vi "BLT Control Panel.vi"() -> ()   [LabVIEW 2018]
uses:
  Type Defs/Sensor Data.ctl
  Type Defs/Boxcar.ctl
panel:
  out "COPV PT":string="-123.37 lbf"
  in  "Data Log Button 2":bool
  out "LOX":dbl(slide) scale=0.0..90.0
  out "current time":timestamp=timestamp(3662240982.153583 s since 1904-01-01)
  out "loadcell 0":string="2.15 On/Off"
  out "loadcell 1":string="-119.97 On/Off"
  out "FUEL MV PT":string="-38.12 "
  out "LOX MV PT":string="-39.05 "
  out "loadcell 2":string="-359.34 On/Off"
  out "90%":string="15.79 °C"
  in  "Box cooler":bool
  out "NewVal":bool
  out "Ready To Fire Flag":bool
  out "Firing State":string[](array[string])=["System Is Not Armed", "  \n", " ", " ", " ", " ", " ", " "]
  in  "Arm Flag":bool
  in  "Sample Rate (secs)":u32=100
  out "Burn Time\nCountdown (secs)":string="0.00"
  out "Boxcar Data":T1={"AI Sensor Data"={"Sensor Array"=[{"Description"="P2 - LOX Tank Pressure", "Last Reading"="-124.93", "Coefs"=[-124.82, 244.17], "Eng Units"="psig"}, {"Description"="P3 - Fuel Tank Pressure", "Last Reading"="-124.93", "Coefs"=[-124.82, 244.17], "Eng Units"="psig"}, {"Description"="P1 - Chamber Pressure", "Last Reading"="-63.48", "Coefs"=[-63.442, 124.53], "Eng Units"="psig"}, {"Description"="Not Used", "Last Reading"="0.00", "Coefs"=[0.0, 0.0], "Eng Units"="psig"}, {"Description"="P5- DOME Reg.", "Last Reading"="-65.08", "Coefs"=[-65.132, -121.72], "Eng Units"="psig"}, {"Description"="Not Use", "Last Reading"="0.00", "Coefs"=[0.0, 0.0], "Eng Units"="psig"}, {"Description"="Load Cell", "Last Reading"="-5.17", "Coefs"=[-8.51, -8297.0], "Eng Units"="lb"}, {"Description"="P7 - Gnd High Pressure", "Last Reading"="-4.44", "Coefs"=[0.0, 10000.0], "Eng Units"="psig"}, {"Description"="High Press PT", "Last Reading"="20.64", "Coefs"=[-546.67, 1244.7], "Eng Units"="psig"}, {"Description"="Dome Reg PT", "Last Reading"="1.90", "Coefs"=[-126.3, 250.5], "Eng Units"="psig"}, {"Description"="FUEL PT", "Last Reading"="1.22", "Coefs"=[-134.15, 250.329], "Eng Units"=""}, {"Description"="LOX PT", "Last Reading"="1.10", "Coefs"=[-129.5, 251.22], "Eng Units"=""}, {"Description"="Chamber PT", "Last Reading"="1.05", "Coefs"=[-63.442, 124.53], "Eng Units"=""}, {"Description"="LOX MV PT", "Last Reading"="-39.05", "Coefs"=[-63.711, 124.59], "Eng Units"=""}, {"Description"="FUEL MV PT", "Last Reading"="-38.12", "Coefs"=[-62.615, 123.79], "Eng Units"=""}, {"Description"="", "Last Reading"="0.00", "Coefs"=[0.0, 0.0], "Eng Units"=""}, {"Description"="", "Last Reading"="2.15", "Coefs"=[1.9166, -16831.0], "Eng Units"="On/Off"}, {"Description"="Load Cell 0", "Last Reading"="-115.96", "Coefs"=[1.9166, -16831.0], "Eng Units"="On/Off"}, {"Description"="Load Cell 1", "Last Reading"="-318.18", "Coefs"=[-0.842, -16966.0], "Eng Units"="On/Off"}, {"Description"="Load Cell 2", "Last Reading"="3.51", "Coefs"=[-0.842, -16966.0], "Eng Units"="On/Off"}, {"Description"="Load Cell 1 - Veh Gross Weight", "Last Reading"="-123.37", "Coefs"=[-122.0, 8333.3], "Eng Units"="lbf"}, {"Description"="Load Cell 2 - - Veh Gross Weight", "Last Reading"="-1.64", "Coefs"=[0.0, 8333.33], "Eng Units"="lbf"}, {"Description"="Extra PT", "Last Reading"="-72.27", "Coefs"=[-72.241, 126.92], "Eng Units"=""}, {"Description"="Not Used", "Last Reading"="0.00", "Coefs"=[0.0, 0.0], "Eng Units"=""}, {"Description"="P6 - GHE Fill Pressure", "Last Reading"="-13651.00", "Coefs"=[-1035.0, 1261.6], "Eng Units"="psi"}, {"Description"="", "Last Reading"="0.00", "Coefs"=[], "Eng Units"=""}, {"Description"="", "Last Reading"="0.00", "Coefs"=[], "Eng Units"=""}, {"Description"="", "Last Reading"="0.00", "Coefs"=[], "Eng Units"=""}, {"Description"="", "Last Reading"="0.00", "Coefs"=[], "Eng Units"=""}, {"Description"="", "Last Reading"="0.00", "Coefs"=[], "Eng Units"=""}, {"Description"="", "Last Reading"="0.00", "Coefs"=[], "Eng Units"=""}, {"Description"="", "Last Reading"="0.00", "Coefs"=[], "Eng Units"=""}]}, "TC Array"=[15.7913203265, 15.7913203265, 15.7913203265, 15.7913203265, 15.7913203265, 15.7913203265, 15.7913203265, 1369.6815, 1369.6815, 1369.6815, 1369.6815, 1369.6815, 1369.6815, 1369.6815]}
  out "?":string="20.64 psig"
  out "Log Refnum":refnum<file>
  out "Log Epoch":u32=140317755
  out "Log Number":i32=426
  in  "Data Log Flag":bool
  out "File Path":path=path "C:/Users/Beach Launch Team/Desktop/EGSE/DATA LOGS/Default Log"
  out "Eng Data & Units":string[](array[string])=["-124.93 psig", "-124.94 psig", "-63.48 psig", "0.00 psig", "-65.08 psig", "0.00 psig", "-5.17 lb", "-4.44 psig", "20.64 psig", "1.90 psig", "1.22 ", "1.10 ", "1.05 ", "-39.05 ", "-38.12 ", "0.00 ", "2.15 On/Off", "-119.97 On/Off", "-359.34 On/Off", "3.51 On/Off", "-123.37 lbf", "-1.64 lbf", "-72.27 ", "0.00 ", "-13651.00 psi", "0.00 ", "0.00 ", "0.00 ", "0.00 ", "0.00 ", "0.00 ", "0.00 "]
  out "TC String Array":string[](array[string])=["15.79 °C", "15.79 °C", "15.79 °C", "15.79 °C", "15.79 °C", "15.79 °C", "15.79 °C", "1369.68 °C", "1369.68 °C", "1369.68 °C", "1369.68 °C", "1369.68 °C", "1369.68 °C", "1369.68 °C"]
  in  "Data Log Button":bool
  in  "Sequence Abort":bool
  out "Igniter Abort":bool
  out "Elapsed Time":u32=10552
  in  "Auto Sequence":bool
  in  "Auto Sequence Flag":bool
  out "Epoch":u32=136578
  out "Countdown (secs)":i32
  in  "MV Open Start":dbl
  in  "Burn Time":dbl=90.0
  in  "Igniter Start":dbl=-6.0
  in  "Countdown":dbl=-10.0
  in  "Igniter Minimum\nTemp (°C)":dbl=60.0
  in  "Auto Switch":bool=TRUE
  out "?":string="1369.68 °C"
  out "Thermometer 2":dbl(slide)=1369.6815 scale=0.0..1000.0
  out "Thermometer":dbl(slide)=1369.6815 scale=0.0..1000.0
  out "Igniter Temp (°C)":string="1369.68 °C"
  out "10%":string="15.79 °C"
  out "50%":string="15.79 °C"
  out "QD Sep Indicator":bool
  out "Liftoff Indicator":bool
  out "MV Closed Ind":bool
  out "MV Open Ind":bool
  out "?":string="1.90 psig"
  out "?":string="-4.44 psig"
  out "Dome Reg PT":string="1.90 psig"
  out "?":string="20.64 psig"
  out "Main Valve PT":string="1.05 "
  out "Fuel PT":string="1.22 "
  in  "High Press":bool
  in  "High Press Vent":bool
  in  "MV Open":bool
  in  "MV Closed":bool
  out "Lox PT":string="1.10 "
  in  "Remote QD Sep":bool
  in  "GHe Fill":bool
  in  "Igniter Pwr":bool
  in  "Dome Reg":bool
  in  "Dome Vent":bool
  in  "Fuel Vent":bool
  in  "LOX Vent":bool
  out "Relay States":bool[](array[boolean])
  in  "stop":bool
  in  "AI Sensor Data":T2={"Sensor Array"=[{"Description"="P2 - LOX Tank Pressure", "Last Reading"="-124.93", "Coefs"=[-124.82, 244.17], "Eng Units"="psig"}, {"Description"="P3 - Fuel Tank Pressure", "Last Reading"="-124.94", "Coefs"=[-124.82, 244.17], "Eng Units"="psig"}, {"Description"="P1 - Chamber Pressure", "Last Reading"="-63.48", "Coefs"=[-63.442, 124.53], "Eng Units"="psig"}, {"Description"="Not Used", "Last Reading"="0.00", "Coefs"=[0.0, 0.0], "Eng Units"="psig"}, {"Description"="P5- DOME Reg.", "Last Reading"="-65.08", "Coefs"=[-65.132, -121.72], "Eng Units"="psig"}, {"Description"="Not Use", "Last Reading"="0.00", "Coefs"=[0.0, 0.0], "Eng Units"="psig"}, {"Description"="Load Cell", "Last Reading"="-5.17", "Coefs"=[-8.51, -8297.0], "Eng Units"="lb"}, {"Description"="P7 - Gnd High Pressure", "Last Reading"="-4.44", "Coefs"=[0.0, 10000.0], "Eng Units"="psig"}, {"Description"="High Press PT", "Last Reading"="20.64", "Coefs"=[-546.67, 1244.7], "Eng Units"="psig"}, {"Description"="Dome Reg PT", "Last Reading"="1.90", "Coefs"=[-126.3, 250.5], "Eng Units"="psig"}, {"Description"="FUEL PT", "Last Reading"="1.22", "Coefs"=[-134.15, 250.329], "Eng Units"=""}, {"Description"="LOX PT", "Last Reading"="1.10", "Coefs"=[-129.5, 251.22], "Eng Units"=""}, {"Description"="Chamber PT", "Last Reading"="1.05", "Coefs"=[-63.442, 124.53], "Eng Units"=""}, {"Description"="LOX MV PT", "Last Reading"="-39.05", "Coefs"=[-63.711, 124.59], "Eng Units"=""}, {"Description"="FUEL MV PT", "Last Reading"="-38.12", "Coefs"=[-62.615, 123.79], "Eng Units"=""}, {"Description"="", "Last Reading"="0.00", "Coefs"=[0.0, 0.0], "Eng Units"=""}, {"Description"="", "Last Reading"="2.15", "Coefs"=[1.9166, -16831.0], "Eng Units"="On/Off"}, {"Description"="Load Cell 0", "Last Reading"="-119.97", "Coefs"=[1.9166, -16831.0], "Eng Units"="On/Off"}, {"Description"="Load Cell 1", "Last Reading"="-359.34", "Coefs"=[-0.842, -16966.0], "Eng Units"="On/Off"}, {"Description"="Load Cell 2", "Last Reading"="3.51", "Coefs"=[-0.842, -16966.0], "Eng Units"="On/Off"}, {"Description"="Load Cell 1 - Veh Gross Weight", "Last Reading"="-123.37", "Coefs"=[-122.0, 8333.3], "Eng Units"="lbf"}, {"Description"="Load Cell 2 - - Veh Gross Weight", "Last Reading"="-1.64", "Coefs"=[0.0, 8333.33], "Eng Units"="lbf"}, {"Description"="Extra PT", "Last Reading"="-72.27", "Coefs"=[-72.241, 126.92], "Eng Units"=""}, {"Description"="Not Used", "Last Reading"="0.00", "Coefs"=[0.0, 0.0], "Eng Units"=""}, {"Description"="P6 - GHE Fill Pressure", "Last Reading"="-13651.00", "Coefs"=[-1035.0, 1261.6], "Eng Units"="psi"}, {"Description"="", "Last Reading"="0.00", "Coefs"=[], "Eng Units"=""}, {"Description"="", "Last Reading"="0.00", "Coefs"=[], "Eng Units"=""}, {"Description"="", "Last Reading"="0.00", "Coefs"=[], "Eng Units"=""}, {"Description"="", "Last Reading"="0.00", "Coefs"=[], "Eng Units"=""}, {"Description"="", "Last Reading"="0.00", "Coefs"=[], "Eng Units"=""}, {"Description"="", "Last Reading"="0.00", "Coefs"=[], "Eng Units"=""}, {"Description"="", "Last Reading"="0.00", "Coefs"=[], "Eng Units"=""}]}
  # "CSULB Launch Team Control System"
  # "Autosequence\n Parameters"
  # "30%"
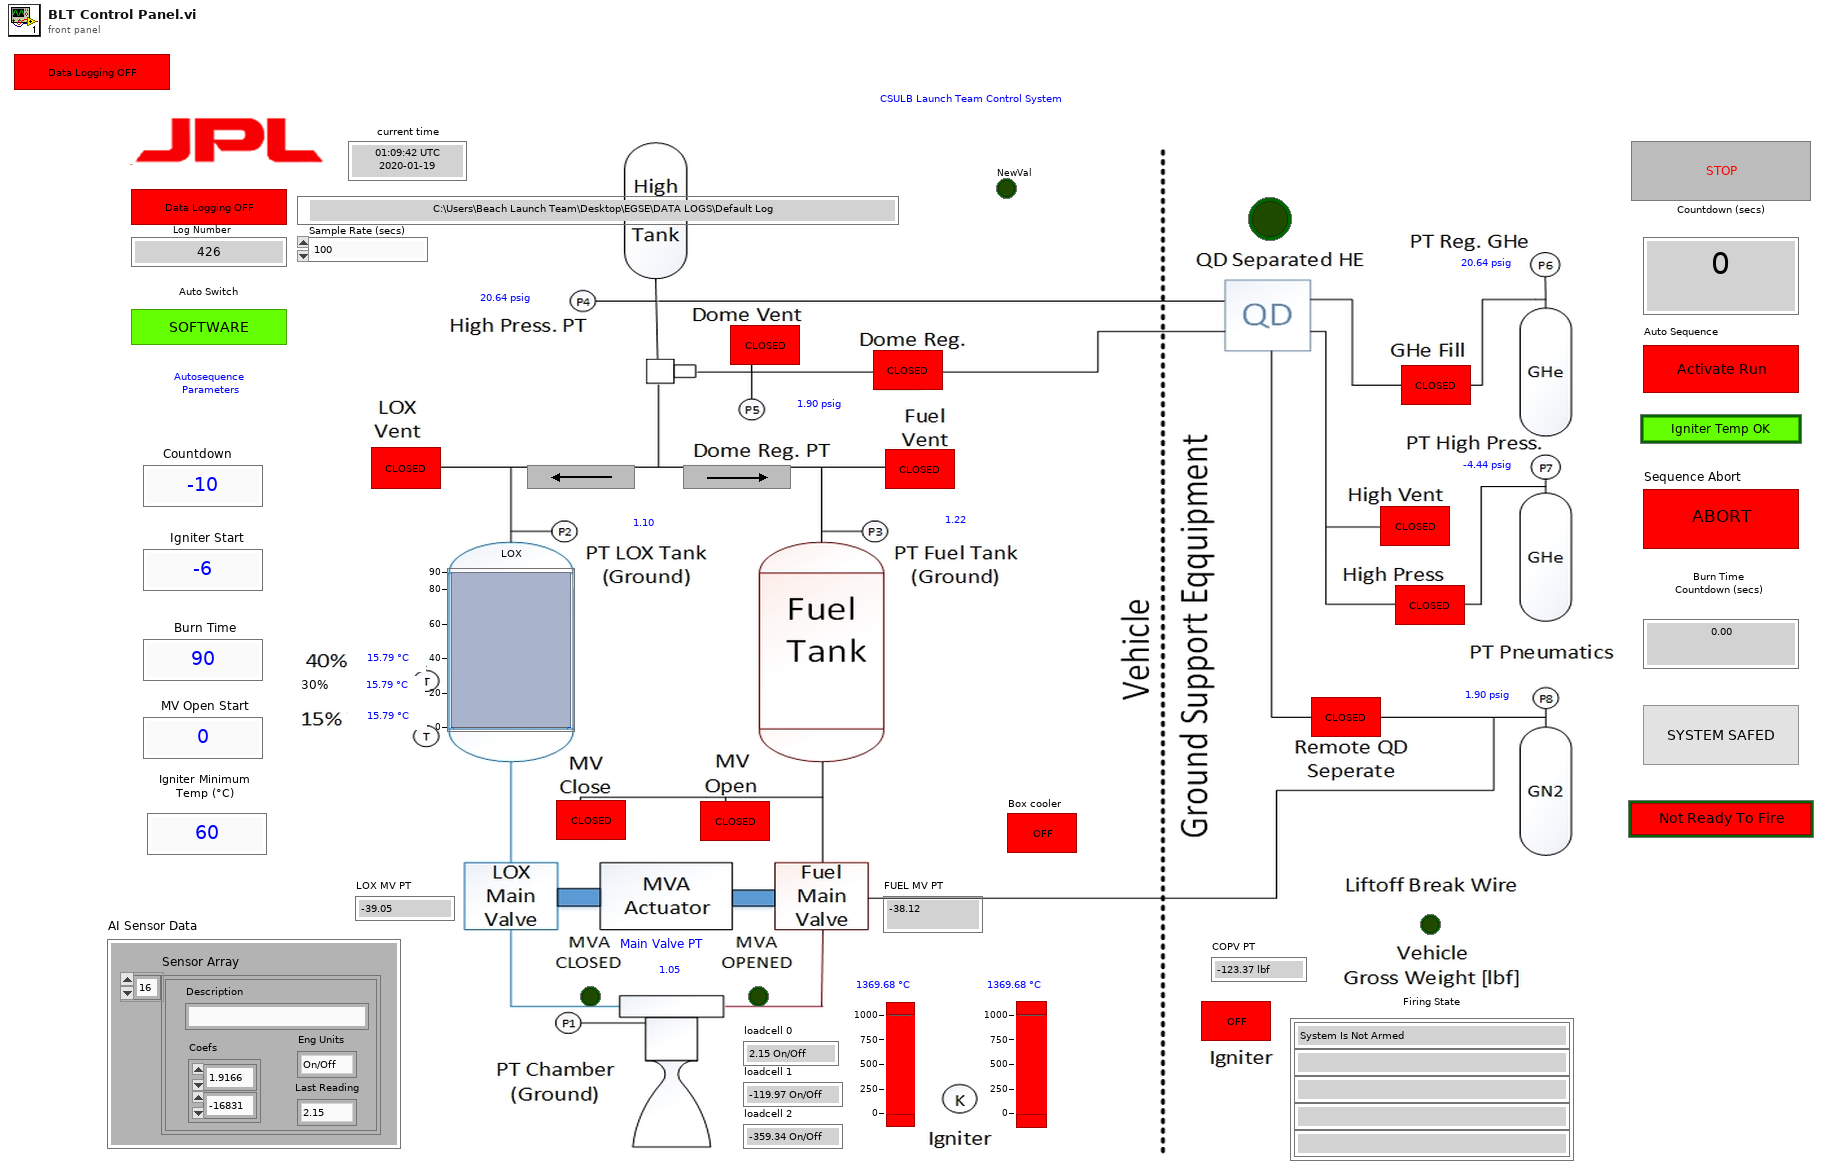
[diagram p1: front panel]
types:
  T1 = typedef "Boxcar.ctl" = cluster{"AI Sensor Data":T2, "TC Array":dbl[]}
  T2 = typedef "Sensor Data.ctl" = cluster{"Sensor Array":cluster{"Description":string, "Last Reading":string, "Coefs":dbl[], "Eng Units":string}[]}
  T3 = enum16{"open", "replace", "create", "open or create", "replace or create", "replace or create with confirmation"}
  T4 = cluster{"Description":string, "Last Reading":string, "Coefs":dbl[], "Eng Units":string}[]
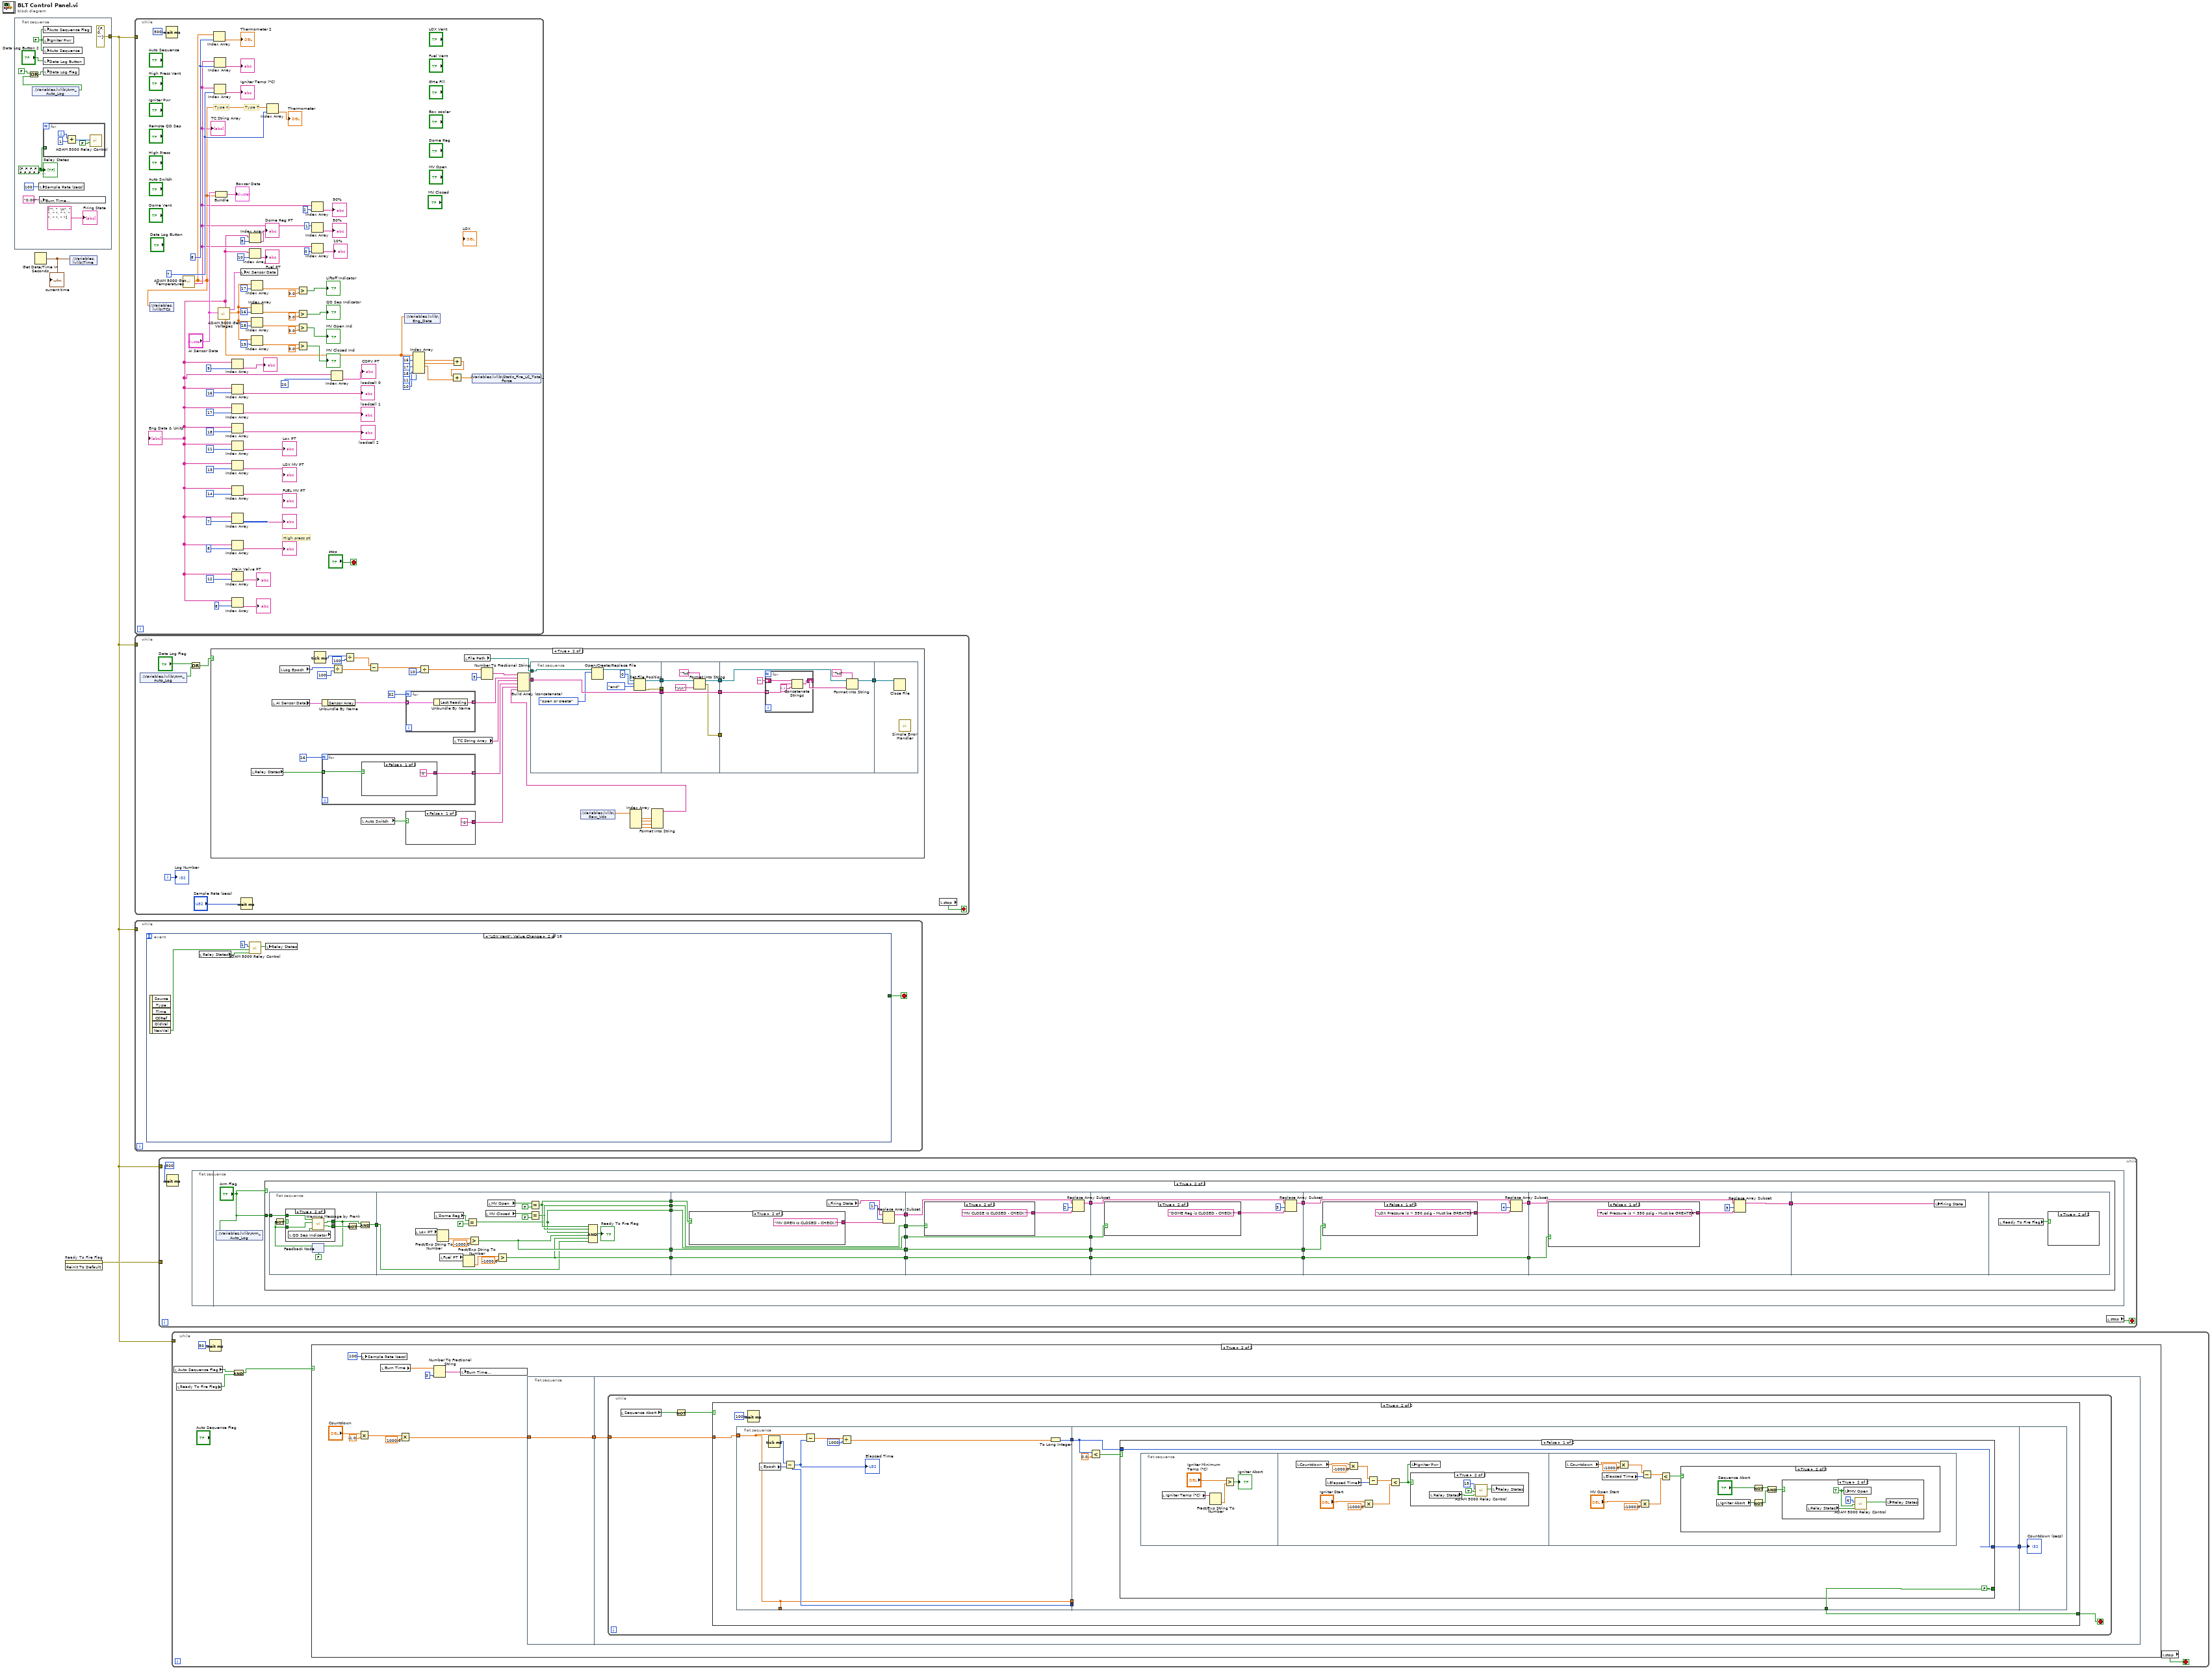
[diagram p0: block diagram]
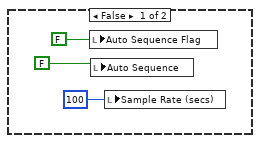
[diagram p2: hidden frame]
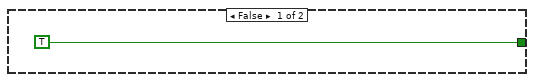
[diagram p3: hidden frame]
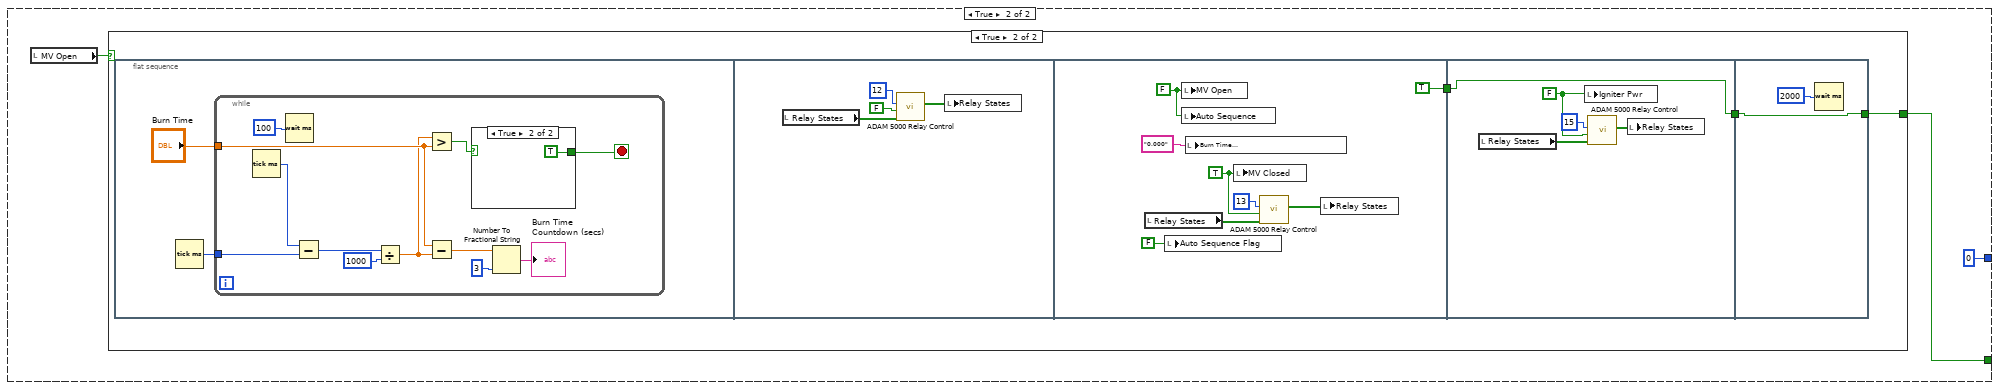
[diagram p7: hidden frame]
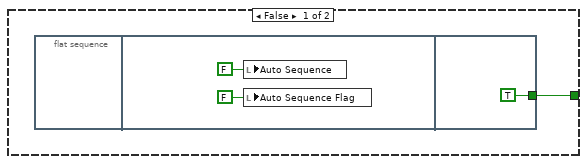
[diagram p8: hidden frame]
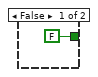
[diagram p9: hidden frame]
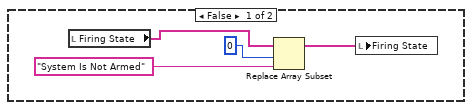
[diagram p10: hidden frame]
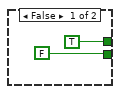
[diagram p11: hidden frame]
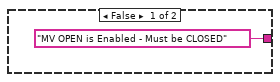
[diagram p12: hidden frame]
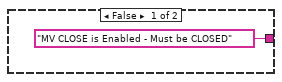
[diagram p13: hidden frame]
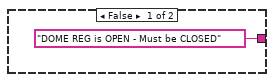
[diagram p14: hidden frame]
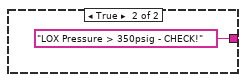
[diagram p15: hidden frame]
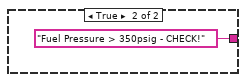
[diagram p16: hidden frame]
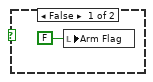
[diagram p17: hidden frame]
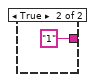
[diagram p19: hidden frame]
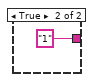
[diagram p20: hidden frame]
diagram:
  n1 = flat-sequence {
    tunnel: [errorcluster {"status"=FALSE, "code"=0, "source"=""} ("error constant")] -> w3
    frame #0 {
      w11 = FALSE ("Auto Sequence Flag")
      w12 = bool[] [FALSE, FALSE, FALSE, FALSE, FALSE, FALSE, FALSE, FALSE, FALSE, FALSE, FALSE, FALSE, FALSE, FALSE, FALSE, FALSE]
      n2 = shared-variable ".\\Variables.lvlib\\Arm_Auto_Log"() -> (w5:bool)  [unwired: 1 in, 1 out]
      n3 = Or(x=FALSE ("Data Lof Flag"), y=w5) -> (x .or. y?=w6:bool)
      n4 = local write "Sample Rate (secs)"(u32 100 ("Sample Rate (secs)")) -> ()
      n5 = local write "Burn Time\nCountdown (secs)"("0.00" ("Burn Time\nCountdown (secs)")) -> ()
      n6 = local write "Auto Sequence Flag"(w11) -> ()
      n7 = local write "Igniter Pwr"(w11) -> ()
      n8 = local write "Auto Sequence"(w11) -> ()
      n9 = local write "Data Log Button"("Data Log Button 2") -> ()
      n10 = local write "Data Log Flag"(w6) -> ()
      n11 = for {
        tunnel: w12 -> [_] mode=indexing
        i -> [w17]
        n12 = Add(x=w17, y=1) -> (x+y=w15:i32)
        n13 = call "ADAM 5000 Relay Control.vi"("State"=FALSE, "Relay # (1=1st relay)"=w15) -> ()  [unwired: 9 in, 1 out]
      }
      "Relay States" <- w12
      "Firing State" <- string[] ["", "  \n", " ", " ", " ", " ", " ", " "]
    }
  }
  n14 = Get Date/Time In Seconds() -> (seconds since 1Jan1904=w1:timestamp)
  "current time" <- w1
  n15 = invoke on="Ready To Fire Flag" class="Bool (strict)" method="Reinit To Default"() -> (error out=w2:errorcluster)  [unwired: 3 in, 2 out]
  n16 = shared-variable ".\\Variables.lvlib\\Time"(w1) -> ()  [unwired: 1 in, 1 out]
  n17 = while {
    tunnel: w3 -> [_]
    stop <- "stop" stop-if-true
    w51 = 8 ("index")
    w54 = 7 ("index")
    # "High press pt"
    # "Type T"
    # "Type K"
    n18 = Wait (ms)(milliseconds to wait=u32 500) -> ()  [unwired: 1 out]
    n19 = call "ADAM 5000 Get Temperatures.vi"() -> ("TC String Array"=w41:string[], "TC Array"=w21:dbl[])  [unwired: 10 in]
    "TC String Array" <- w41
    n20 = shared-variable ".\\Variables.lvlib\\TCs"(w21) -> ()  [unwired: 1 in, 1 out]
    n21 = Index Array(array=w21, index=w51) -> (element=→"Thermometer 2":dbl)
    n22 = Index Array(array=w41, index=w51) -> (element=→"?":string)
    n23 = Index Array(array=w41, index=w54) -> (element=→"Igniter Temp (°C)":string)
    n24 = Bundle("AI Sensor Data"="AI Sensor Data", "TC Array"=w21) -> (→"Boxcar Data":cluster{"AI Sensor Data":T2, "TC Array":dbl[]})  [unwired: 1 in]
    n25 = call "ADAM 5000 Get Voltages.vi"("AI Sensor Data"="AI Sensor Data") -> ("Master Raw Data Vdc"=w60:dbl[], "AI Sensor Data Out"=w91:T2, "Eng Data"=w22:dbl[], "Eng Data & Units"=w18:string[])  [unwired: 5 in, 2 out]
    "Eng Data & Units" <- w18
    n26 = Index Array(array=w18, index=9) -> (element=→"?":string)
    n27 = Index Array(array=w18, index=16) -> (element=→"loadcell 0":string)
    n28 = Index Array(array=w18, index=17) -> (element=→"loadcell 1":string)
    n29 = Index Array(array=w18, index=18) -> (element=→"loadcell 2":string)
    n30 = Index Array(array=w18, index=11) -> (element=→"Lox PT":string)
    n31 = Index Array(array=w18, index=13) -> (element=→"LOX MV PT":string)
    n32 = Index Array(array=w18, index=14) -> (element=→"FUEL MV PT":string)
    n33 = Index Array(array=w18, index=7) -> (element=→"?":string)
    n34 = Index Array(array=w18, index=8) -> (element=→"?":string)
    n35 = Index Array(array=w18, index=12) -> (element=→"Main Valve PT":string)
    n36 = Index Array(array=w18, index=8) -> (element=→"?":string)
    n37 = local write "AI Sensor Data"(w91) -> ()
    n38 = Index Array(array=w18, index=9) -> (element=→"Dome Reg PT":string)
    n39 = Index Array(array=w18, index=10) -> (element=→"Fuel PT":string)
    n40 = Index Array(array=w60, index=17) -> (element=w67:dbl)
    n41 = Index Array(array=w60, index=16) -> (element=w62:dbl)
    n42 = Index Array(array=w60, index=18) -> (element=w75:dbl)
    n43 = Index Array(array=w60, index=19) -> (element=w71:dbl)
    n44 = Index Array(array=w21, index=w54) -> (element=→"Thermometer":dbl)
    n45 = Greater?(x=w67, y=3.0) -> (0:→"Liftoff Indicator":bool)
    n46 = Greater?(x=w62, y=3.0) -> (0:→"QD Sep Indicator":bool)
    n47 = Greater?(x=w75, y=3.0) -> (0:→"MV Open Ind":bool)
    n48 = Greater?(x=w71, y=3.0) -> (0:→"MV Closed Ind":bool)
    n49 = Index Array(array=w41, index=2) -> (element=→"90%":string)
    n50 = Index Array(array=w41, index=1) -> (element=→"50%":string)
    n51 = Index Array(array=w41, index=0) -> (element=→"10%":string)
    n52 = Index Array(array=w18, index=20) -> (element=→"COPV PT":string)
    n53 = shared-variable ".\\Variables.lvlib\\Eng_Data"(w22) -> ()  [unwired: 1 in, 1 out]
    n54 = Index Array(array=w22, index #1=16 ("index"), index #2=17 ("index"), index #3=18 ("index"), index #4=11 ("index"), index #5=10 ("index")) -> (element #1=w29:dbl, element #2=w28:dbl, element #3=w26:dbl)  [unwired: 2 out]
    n55 = Add(x=w29, y=w28) -> (x+y=w27:dbl)
    n56 = Add(x=w27, y=w26) -> (x+y=w25:dbl)
    n57 = shared-variable ".\\Variables.lvlib\\Static_Fire_LC_Total_Force"(w25) -> ()  [unwired: 1 in, 1 out]
  }
  n58 = while {
    tunnel: w3 -> [_]
    i -> [w98]
    stop <- w99 stop-if-true
    n59 = shared-variable ".\\Variables.lvlib\\Arm_Auto_Log"() -> (w95:bool)  [unwired: 1 in, 1 out]
    n60 = Or(x="Data Log Flag", y=w95) -> (x .or. y?=w94:bool)
    n61 = case shown="True" w94 {
      frame False {
      }
      frame True {
        n62 = local read "Relay States"() -> (w133:bool[])
        n63 = local read "AI Sensor Data"() -> (w135:T2)
        n64 = local read "Log Epoch"() -> (w110:u32)
        n65 = Tick Count (ms)() -> (millisecond timer value=w113:u32)
        n66 = Unbundle By Name(w135) -> ("Sensor Array"=w134:T4)
        n67 = for {
          N: 16 -> [_]
          tunnel: w133 -> [w164] mode=indexing
          tunnel: [w163] -> w129 mode=indexing
          n68 = case shown="False" w164 {
            tunnel: ["0" "1"] -> w163
            frame False {
            }
            frame True {
            }
          }
        }
        n69 = Divide(x=w110, y=u32 100) -> (x/y=w108:dbl)
        n70 = Divide(x=w113, y=u32 100) -> (x/y=w111:dbl)
        n71 = local read "Auto Switch"() -> (w132:bool)
        n72 = Subtract(x=w111, y=w108) -> (x-y=w127:dbl)
        n73 = for {
          N: 32 -> [_]
          tunnel: w134 -> [w168] mode=indexing
          tunnel: [w167] -> w131 mode=indexing
          n74 = Unbundle By Name(w168) -> ("Last Reading"=w167:string)
        }
        n75 = case shown="False" w132 {
          tunnel: ["0" "1"] -> w128
          frame False {
          }
          frame True {
          }
        }
        n76 = Divide(x=w127, y=u32 10) -> (x/y=w125:dbl)
        n77 = local read "TC String Array"() -> (w130:string[])
        n78 = local read "File Path"() -> (w122:path)
        n79 = Number To Fractional String(number=w125, precision (6)=i16 3) -> (F-format string=w123:string)  [unwired: 2 in]
        n80 = flat-sequence {
          tunnel: w121 -> [w143]
          tunnel: w122 -> [w137]
          tunnel: [w143] -> w119
          tunnel: [w139] -> w116
          tunnel: [w136] -> w101
          tunnel: [w145] -> w120
          tunnel: w119 -> [w149]
          tunnel: [w149] -> w118
          tunnel: w116 -> [w146]
          tunnel: w101 -> [_]
          tunnel: [w144] -> w100
          tunnel: w120 -> [w152]
          tunnel: w118 -> [w155]
          tunnel: [w150] -> w117
          tunnel: w100 -> [_]
          tunnel: w117 -> [w160]
          frame #0 {
            n81 = Open/Create/Replace File(file path (use dialog)=w137, operation (0:open)=T3."open or create") -> (refnum out=w142:refnum<file>)  [unwired: 4 in, 2 out]
            n82 = Set File Position(offset (in bytes) (0)=i64 0, refnum=w142, from (0:start)=enum16{"start", "end", "current"}."end") -> (refnum out=w139:refnum<file>, error out=w136:errorcluster)  [unwired: 1 in]
          }
          frame #1 {
            n83 = Format Into String(format string="%s", initial string=w146, "\r\n") -> (resulting string=w145:refnum<file>, error out=w144:errorcluster)  [unwired: 1 in]
          }
          frame #2 {
            n84 = for {
              shift-right: [w157] -> w151
              shift-left: "" -> [w156]
              tunnel: w155 -> [w159] mode=indexing
              n85 = Concatenate Strings(w156, w159, "," ("string")) -> (w157:string)
            }
            n86 = Format Into String(format string="%s", initial string=w152, w151) -> (resulting string=w150:refnum<file>)  [unwired: 1 in, 1 out]
          }
          frame #3 {
            n87 = Close File(refnum=w160) -> ()  [unwired: 1 in, 2 out]
            n88 = call <vilib>:"Simple Error Handler.vi"() -> ()  [unwired: 5 in, 5 out]
          }
        }
        n89 = shared-variable ".\\Variables.lvlib\\Raw_Vdc"() -> (w107:dbl[])  [unwired: 1 in, 1 out]
        n90 = Index Array(array=w107) -> (element #1=w106:dbl, element #2=w105:dbl, element #3=w103:dbl, element #4=w102:dbl)  [unwired: 4 in]
        n91 = Format Into String(w106, w105, w103, w102) -> (resulting string=w104:string)  [unwired: 3 in, 1 out]
        n92 = Build Array (concatenate)(w123, w131, w130, w129, w128, w104) -> (w121:string[])
      }
    }
    n93 = Wait (ms)(milliseconds to wait="Sample Rate (secs)") -> ()  [unwired: 1 out]
    n94 = local read "stop"() -> (w99:bool)
    "Log Number" <- w98
  }
  n95 = while {
    tunnel: w3 -> [_]
    stop <- w169 stop-if-true
    n96 = event shown="[1] \"LOX Vent\": Value Change" {
      selector: _ -> [_ _ _ _ _ _ _ _ _ _ _ _ _ _ _ _ _ _]
      dyn-events: _ -> [_ _ _ _ _ _ _ _ _ _ _ _ _ _ _ _ _ _]
      timeout: _ -> [_ _ _ _ _ _ _ _ _ _ _ _ _ _ _ _ _ _]
      tunnel: [_ _ _ _ _ _ _ _ w198 _ _ _ _ _ _ _ _ _] -> w169
      event Timeout {
        n97 = event-data() -> ()  [unwired: 1 in, 3 out]
      }
      event "LOX Vent": Value Change {
        n98 = event-data() -> ("NewVal"=w172:bool)  [unwired: 1 in, 5 out]
        n99 = local read "Relay States"() -> (w171:bool[])
        n100 = call "ADAM 5000 Relay Control.vi"("Relay States IN"=w171, "State"=w172, "Relay # (1=1st relay)"=1) -> ("Relay States OUT"=w170:bool[])  [unwired: 8 in]
        n101 = local write "Relay States"(w170) -> ()
      }
      event "Fuel Vent": Value Change {
        n102 = event-data() -> ("NewVal"=w174:bool)  [unwired: 1 in, 5 out]
        n103 = local read "Relay States"() -> (w176:bool[])
        n104 = call "ADAM 5000 Relay Control.vi"("Relay States IN"=w176, "State"=w174, "Relay # (1=1st relay)"=2) -> ("Relay States OUT"=w175:bool[])  [unwired: 8 in]
        n105 = local write "Relay States"(w175) -> ()
      }
      event "Dome Vent": Value Change {
        n106 = event-data() -> ("NewVal"=w178:bool)  [unwired: 1 in, 5 out]
        n107 = local read "Relay States"() -> (w180:bool[])
        n108 = call "ADAM 5000 Relay Control.vi"("Relay States IN"=w180, "State"=w178, "Relay # (1=1st relay)"=3) -> ("Relay States OUT"=w179:bool[])  [unwired: 8 in]
        n109 = local write "Relay States"(w179) -> ()
      }
      event "Dome Reg": Value Change {
        n110 = event-data() -> ("NewVal"=w182:bool)  [unwired: 1 in, 5 out]
        n111 = local read "Relay States"() -> (w184:bool[])
        n112 = call "ADAM 5000 Relay Control.vi"("Relay States IN"=w184, "State"=w182, "Relay # (1=1st relay)"=4) -> ("Relay States OUT"=w183:bool[])  [unwired: 8 in]
        n113 = local write "Relay States"(w183) -> ()
      }
      event "Igniter Pwr": Value Change {
        n114 = event-data() -> ("NewVal"=w186:bool)  [unwired: 1 in, 5 out]
        n115 = local read "Relay States"() -> (w188:bool[])
        n116 = call "ADAM 5000 Relay Control.vi"("Relay States IN"=w188, "State"=w186, "Relay # (1=1st relay)"=15) -> ("Relay States OUT"=w187:bool[])  [unwired: 8 in]
        n117 = local write "Relay States"(w187) -> ()
      }
      event "GHe Fill": Value Change {
        n118 = event-data() -> ("NewVal"=w190:bool)  [unwired: 1 in, 5 out]
        n119 = local read "Relay States"() -> (w192:bool[])
        n120 = call "ADAM 5000 Relay Control.vi"("Relay States IN"=w192, "State"=w190, "Relay # (1=1st relay)"=12) -> ("Relay States OUT"=w191:bool[])  [unwired: 8 in]
        n121 = local write "Relay States"(w191) -> ()
      }
      event "Remote QD Sep": Value Change {
        n122 = event-data() -> ("NewVal"=w194:bool)  [unwired: 1 in, 5 out]
        n123 = local read "Relay States"() -> (w196:bool[])
        n124 = call "ADAM 5000 Relay Control.vi"("Relay States IN"=w196, "State"=w194, "Relay # (1=1st relay)"=11) -> ("Relay States OUT"=w195:bool[])  [unwired: 8 in]
        n125 = local write "Relay States"(w195) -> ()
      }
      event "stop": Value Change {
        n126 = event-data() -> ()  [unwired: 1 in, 6 out]
        n127 = flat-sequence {
          tunnel: [TRUE] -> w198
          frame #0 {
            n128 = Wait (ms)(milliseconds to wait=u32 2000) -> ()  [unwired: 1 out]
          }
          frame #1 {
          }
        }
      }
      event "MV Closed": Value Change {
        n129 = event-data() -> ("NewVal"=w201:bool)  [unwired: 1 in, 5 out]
        n130 = local read "Relay States"() -> (w203:bool[])
        n131 = call "ADAM 5000 Relay Control.vi"("Relay States IN"=w203, "State"=w201, "Relay # (1=1st relay)"=5) -> ("Relay States OUT"=w202:bool[])  [unwired: 8 in]
        n132 = local write "Relay States"(w202) -> ()
      }
      event "High Press Vent": Value Change {
        n133 = event-data() -> ("NewVal"=w205:bool)  [unwired: 1 in, 5 out]
        n134 = local read "Relay States"() -> (w207:bool[])
        n135 = call "ADAM 5000 Relay Control.vi"("Relay States IN"=w207, "State"=w205, "Relay # (1=1st relay)"=10) -> ("Relay States OUT"=w206:bool[])  [unwired: 8 in]
        n136 = local write "Relay States"(w206) -> ()
      }
      event "High Press": Value Change {
        n137 = event-data() -> ("NewVal"=w209:bool)  [unwired: 1 in, 5 out]
        n138 = local read "Relay States"() -> (w211:bool[])
        n139 = call "ADAM 5000 Relay Control.vi"("Relay States IN"=w211, "State"=w209, "Relay # (1=1st relay)"=9) -> ("Relay States OUT"=w210:bool[])  [unwired: 8 in]
        n140 = local write "Relay States"(w210) -> ()
      }
      event "Auto Switch": Value Change {
        n141 = event-data() -> ("NewVal"=w214:bool)  [unwired: 1 in, 5 out]
        n142 = call "Control ETH008 Relay.vi"("On/Off"=w214, "Relay Number"=1) -> ()  [unwired: 10 in]
      }
      event "Auto Sequence": Value Change {
        w216 = TRUE ("Auto Sequence Flag")
        n143 = event-data() -> ()  [unwired: 1 in, 6 out]
        n144 = Tick Count (ms)() -> (millisecond timer value=→"Epoch":u32)
        n145 = local write "Auto Sequence Flag"(w216) -> ()
        n146 = local write "Auto Sequence"(w216) -> ()
      }
      event "Sequence Abort": Value Change {
        n147 = event-data() -> ()  [unwired: 1 in, 6 out]
        n148 = flat-sequence {
          frame #0 {
            w217 = FALSE ("Auto Sequence Flag")
            n149 = local write "Auto Sequence Flag"(w217) -> ()
            n150 = local write "Igniter Pwr"(w217) -> ()
            n151 = local write "Auto Sequence"(w217) -> ()
          }
          frame #1 {
            n152 = for {
              tunnel: bool[] [FALSE, FALSE, FALSE, FALSE, FALSE, FALSE, FALSE, FALSE, FALSE, FALSE, FALSE, FALSE, FALSE, FALSE, FALSE, FALSE] -> [_] mode=indexing
              i -> [w222]
              n153 = Add(x=w222, y=1) -> (x+y=w220:i32)
              n154 = call "ADAM 5000 Relay Control.vi"("State"=FALSE, "Relay # (1=1st relay)"=w220) -> ()  [unwired: 9 in, 1 out]
            }
          }
        }
      }
      event "Data Log Button": Value Change {
        n155 = event-data() -> ("NewVal"=w223:bool)  [unwired: 1 in, 5 out]
        n156 = case shown="True" w223 {
          frame False {
            n157 = local write "Data Log Flag"(FALSE ("Data Lof Flag")) -> ()
            n158 = local write "Data Log Flag"(FALSE ("Data Lof Flag")) -> ()
            n159 = local write "Data Log Flag"(FALSE ("Data Lof Flag")) -> ()
            n160 = local write "Data Log Flag"(FALSE ("Data Lof Flag")) -> ()
            n161 = local write "Data Log Flag"(FALSE ("Data Lof Flag")) -> ()
            n162 = local write "Data Log Flag"(FALSE ("Data Lof Flag")) -> ()
            n163 = local write "Data Log Flag"(FALSE ("Data Lof Flag")) -> ()
            n164 = local write "Data Log Flag"(FALSE ("Data Lof Flag")) -> ()
            n165 = local write "Data Log Flag"(FALSE ("Data Lof Flag")) -> ()
            n166 = local write "Data Log Flag"(FALSE ("Data Lof Flag")) -> ()
            n167 = local write "Data Log Flag"(FALSE ("Data Lof Flag")) -> ()
          }
          frame True {
            n168 = flat-sequence {
              frame #0 {
                n169 = Tick Count (ms)() -> (millisecond timer value=→"Log Epoch":u32)
                n170 = for {
                  N: 14 -> [_]
                  tunnel: [w267] -> w246 mode=indexing
                  i -> [w266]
                  n171 = Add(x=w266, y=1) -> (x+y=w264:i32)
                  n172 = Number To Fractional String(number=w264, precision (6)=i16 0) -> (F-format string=w268:string)  [unwired: 2 in]
                  n173 = Concatenate Strings("TC", w268) -> (w267:string)
                }
                n174 = for {
                  N: 16 -> [_]
                  tunnel: [w260] -> w245 mode=indexing
                  i -> [w259]
                  n175 = Add(x=w259, y=1) -> (x+y=w257:i32)
                  n176 = Number To Fractional String(number=w257, precision (6)=i16 0) -> (F-format string=w261:string)  [unwired: 2 in]
                  n177 = Concatenate Strings("Relay", w261) -> (w260:string)
                }
                n178 = local read "AI Sensor Data"() -> (w252:T2)
                n179 = Unbundle By Name(w252) -> ("Sensor Array"=w251:T4)
                n180 = for {
                  tunnel: w251 -> [w272] mode=indexing
                  tunnel: [w271] -> w249 mode=indexing
                  n181 = Unbundle By Name(w272) -> ("Description"=w271:string)
                }
                n182 = Build Array (concatenate)("Time (s)", w249, w246, w245, "Manual/Auto (1=Auto)") -> (w241:string[])
                n183 = Open/Create/Replace File(operation (0:open)=T3."open or create") -> (refnum out=w235:refnum<file>)  [unwired: 5 in, 2 out]
                "Log Refnum" <- w235
                n184 = for {
                  shift-right: [w254] -> w239
                  shift-left: "" -> [w253]
                  tunnel: w241 -> [w256] mode=indexing
                  n185 = Concatenate Strings(w253, w256, "," ("string")) -> (w254:string)
                }
                n186 = Refnum to Path(1:w235) -> (0:w238:path)
                "File Path" <- w238
                n187 = Format Into String(format string="%s", initial string=w235, w239) -> (resulting string=w237:refnum<file>)  [unwired: 1 in, 1 out]
                n188 = local write "File Path"(w238) -> ()
                n189 = Close File(refnum=w237) -> ()  [unwired: 1 in, 2 out]
              }
              frame #1 {
                n190 = Wait (ms)(milliseconds to wait=u32 10) -> ()  [unwired: 1 out]
              }
              frame #2 {
                n191 = local write "Data Log Flag"(TRUE ("Data Lof Flag")) -> ()
              }
            }
          }
        }
      }
      event "MV Open": Value Change {
        n192 = event-data() -> ("NewVal"=w278:bool)  [unwired: 1 in, 5 out]
        "NewVal" <- w278
        n193 = local read "Relay States"() -> (w276:bool[])
        n194 = call "ADAM 5000 Relay Control.vi"("Relay States IN"=w276, "State"=w278, "Relay # (1=1st relay)"=6) -> ("Relay States OUT"=w277:bool[])  [unwired: 8 in]
        n195 = local write "Relay States"(w277) -> ()
      }
      event "Box cooler": Value Change {
        n196 = event-data() -> ("NewVal"=w279:bool)  [unwired: 1 in, 5 out]
        n197 = local read "Relay States"() -> (w281:bool[])
        n198 = call "ADAM 5000 Relay Control.vi"("Relay States IN"=w281, "State"=w279, "Relay # (1=1st relay)"=3) -> ("Relay States OUT"=w282:bool[])  [unwired: 8 in]
        n199 = local write "Relay States"(w282) -> ()
      }
    }
  }
  n200 = while {
    tunnel: w3 -> [_]
    tunnel: w2 -> [_]
    stop <- w283 stop-if-true
    n201 = Wait (ms)(milliseconds to wait=u32 500) -> ()  [unwired: 1 out]
    n202 = flat-sequence {
      frame #0 {
      }
      frame #1 {
        n203 = shared-variable ".\\Variables.lvlib\\Arm_Auto_Log"("Arm Flag") -> ()  [unwired: 1 in, 1 out]
        n204 = case shown="True" "Arm Flag" {
          tunnel: "Arm Flag" -> [_ w291]
          frame False {
            n205 = local read "Firing State"() -> (w289:string[])
            n206 = Replace Array Subset(array=w289, new element="System Is Not Armed" ("new element/subarray"), index=0) -> (w286:string[])
            n207 = local write "Firing State"(w286) -> ()
          }
          frame True {
            n208 = flat-sequence {
              tunnel: w291 -> [w319]
              tunnel: [w312] -> w290
              tunnel: [w333] -> w311
              tunnel: [w332] -> w309
              tunnel: [w331] -> w305
              tunnel: [w330] -> w299
              tunnel: [w329] -> w294
              tunnel: w290 -> [w327]
              tunnel: w311 -> [w354]
              tunnel: [w350] -> w310
              tunnel: w309 -> [w350]
              tunnel: [w349] -> w308
              tunnel: [w348] -> w306
              tunnel: w305 -> [w348]
              tunnel: [w347] -> w300
              tunnel: w299 -> [w347]
              tunnel: [w346] -> w295
              tunnel: w294 -> [w346]
              tunnel: w310 -> [w362]
              tunnel: w308 -> [w361]
              tunnel: [w360] -> w307
              tunnel: w306 -> [w360]
              tunnel: [w359] -> w304
              tunnel: [w358] -> w301
              tunnel: w300 -> [w358]
              tunnel: [w357] -> w296
              tunnel: w295 -> [w357]
              tunnel: w307 -> [w371]
              tunnel: w304 -> [w370]
              tunnel: [w369] -> w303
              tunnel: [w368] -> w302
              tunnel: w301 -> [w368]
              tunnel: [w367] -> w297
              tunnel: w296 -> [w367]
              tunnel: w303 -> [w379]
              tunnel: w302 -> [w378]
              tunnel: [w377] -> w298
              tunnel: w297 -> [w377]
              tunnel: [w376] -> w293
              tunnel: w298 -> [w386]
              tunnel: w293 -> [w385]
              tunnel: [w384] -> w292
              tunnel: w292 -> [w391]
              frame #0 {
                n209 = feedback #1(FALSE) -> (w313:bool)
                n210 = Not(x=w313) -> (.not. x?=w318:bool)
                n211 = case shown="True" w318 {
                  tunnel: w319 -> [_ w326]
                  tunnel: [FALSE w325] -> w316
                  tunnel: [TRUE w324] -> w315
                  tunnel: w313 -> [_ w323]
                  frame False {
                  }
                  frame True {
                    n212 = local read "QD Sep Indicator"() -> (w322:bool)
                    n213 = call "Warning Message by Frank.vi"("Contiuous"=w322, "ok?"=w323, "Arm Flag"=w326) -> ("super cancel"=w325:bool, "super ok"=w324:bool)  [unwired: 6 in, 1 out]
                  }
                }
                n214 = feedback-in #1(w315) -> ()
                n215 = Not(x=w316) -> (.not. x?=w317:bool)
                n216 = And(x=w315, y=w317) -> (x .and. y?=w312:bool)
              }
              frame #1 {
                n217 = local read "Lox PT"() -> (w339:string)
                n218 = local read "Dome Reg"() -> (w341:bool)
                n219 = Fract/Exp String To Number(string=w339) -> (number=w338:dbl)  [unwired: 3 in, 1 out]
                n220 = local read "Fuel PT"() -> (w334:string)
                n221 = Fract/Exp String To Number(string=w334) -> (number=w335:dbl)  [unwired: 3 in, 1 out]
                n222 = Equal?(x=w341, y=FALSE) -> (x = y?=w331:bool)
                n223 = Greater?(x=w338, y=-1000.0) -> (0:w330:bool)
                n224 = local read "MV Closed"() -> (w342:bool)
                n225 = local read "MV Open"() -> (w345:bool)
                n226 = Greater?(x=w335, y=-1000.0) -> (0:w329:bool)
                n227 = Equal?(x=w345, y=FALSE) -> (x = y?=w333:bool)
                n228 = Equal?(x=w342, y=FALSE) -> (x = y?=w332:bool)
                n229 = Compound Arithmetic op=AND(w333, w332, w331, w330, w329, w327) -> (→"Ready To Fire Flag":bool)
              }
              frame #2 {
                n230 = case shown="True" w354 {
                  tunnel: ["MV OPEN is Enabled - Must be CLOSED" "MV OPEN Is CLOSED - CHECK!"] -> w351
                  frame False {
                  }
                  frame True {
                  }
                }
                n231 = local read "Firing State"() -> (w353:string[])
                n232 = Replace Array Subset(array=w353, new element=w351, index=1) -> (w349:string[])
              }
              frame #3 {
                n233 = case shown="True" w362 {
                  tunnel: ["MV CLOSE is Enabled - Must be CLOSED" "MV CLOSE Is CLOSED - CHECK!"] -> w364
                  frame False {
                  }
                  frame True {
                  }
                }
                n234 = Replace Array Subset(array=w361, new element=w364, index=2) -> (w359:string[])
              }
              frame #4 {
                n235 = case shown="True" w371 {
                  tunnel: ["DOME REG is OPEN - Must be CLOSED" "DOME Reg is CLOSED - CHECK!"] -> w372
                  frame False {
                  }
                  frame True {
                  }
                }
                n236 = Replace Array Subset(array=w370, new element=w372, index=3) -> (w369:string[])
              }
              frame #5 {
                n237 = case shown="False" w378 {
                  tunnel: ["LOX Pressure is < 350 psig - Must be GREATER" "LOX Pressure > 350psig - CHECK!"] -> w381
                  frame False {
                  }
                  frame True {
                  }
                }
                n238 = Replace Array Subset(array=w379, new element=w381, index=4) -> (w376:string[])
              }
              frame #6 {
                n239 = case shown="False" w386 {
                  tunnel: ["Fuel Pressure is < 350 psig - Must be GREATER" "Fuel Pressure > 350psig - CHECK!"] -> w387
                  frame False {
                  }
                  frame True {
                  }
                }
                n240 = Replace Array Subset(array=w385, new element=w387, index=5) -> (w384:string[])
              }
              frame #7 {
                n241 = local write "Firing State"(w391) -> ()
              }
              frame #8 {
                n242 = local read "Ready To Fire Flag"() -> (w392:bool)
                n243 = case shown="True" w392 {
                  frame False {
                    n244 = local write "Arm Flag"(FALSE ("Arm Flag")) -> ()
                  }
                  frame True {
                  }
                }
              }
            }
          }
        }
      }
    }
    n245 = local read "stop"() -> (w283:bool)
  }
  n246 = while {
    tunnel: w3 -> [_]
    stop <- w398 stop-if-true
    n247 = local read "Auto Sequence Flag"() -> (w395:bool)
    n248 = local read "Ready To Fire Flag"() -> (w396:bool)
    n249 = Wait (ms)(milliseconds to wait=u32 50) -> ()  [unwired: 1 out]
    n250 = And(x=w395, y=w396) -> (x .and. y?=w394:bool)
    n251 = case shown="True" w394 {
      frame False {
        n252 = local write "Auto Sequence Flag"(FALSE ("Auto Sequence Flag")) -> ()
        n253 = local write "Auto Sequence"(FALSE ("Auto Sequence Flag")) -> ()
        n254 = local write "Sample Rate (secs)"(u32 100 ("Sample Rate (secs)")) -> ()
      }
      frame True {
        n255 = Multiply(x="Countdown", y=-1.0) -> (x*y=w406:dbl)
        n256 = local write "Sample Rate (secs)"(u32 100 ("Sample Rate (secs)")) -> ()
        n257 = local read "Burn Time"() -> (w405:dbl)
        n258 = Multiply(x=w406, y=1000.0) -> (x*y=w410:dbl)
        n259 = Number To Fractional String(number=w405, precision (6)=i16 3) -> (F-format string=w403:string)  [unwired: 2 in]
        n260 = local write "Burn Time\nCountdown (secs)"(w403) -> ()
        n261 = flat-sequence {
          tunnel: w410 -> [w412]
          tunnel: [w412] -> w409
          tunnel: w409 -> [w413]
          frame #0 {
          }
          frame #1 {
            n262 = while {
              tunnel: w413 -> [w417]
              stop <- w414 stop-if-true
              n263 = local read "Sequence Abort"() -> (w416:bool)
              n264 = Not(x=w416) -> (.not. x?=w415:bool)
              n265 = case shown="True" w415 {
                tunnel: w417 -> [_ w421]
                tunnel: [TRUE w419] -> w414
                frame False {
                }
                frame True {
                  n266 = flat-sequence {
                    tunnel: [w428] -> _
                    tunnel: w421 -> [w428]
                    tunnel: [w429] -> w425
                    tunnel: [w428] -> w424
                    tunnel: [w426] -> w423
                    tunnel: w425 -> [_]
                    tunnel: w424 -> [_]
                    tunnel: w423 -> [w435]
                    tunnel: [w437] -> w419
                    tunnel: [w434] -> w422
                    tunnel: w422 -> [w521]
                    frame #0 {
                      n267 = local read "Epoch"() -> (w427:u32)
                      n268 = Tick Count (ms)() -> (millisecond timer value=w433:u32)
                      n269 = Subtract(x=w433, y=w427) -> (x-y=w429:u32)
                      "Elapsed Time" <- w429
                      n270 = Subtract(x=w428, y=w429) -> (x-y=w430:dbl)
                      n271 = Divide(x=w430, y=u32 1000) -> (x/y=w431:dbl)
                      n272 = To Long Integer(number=w431) -> (32bit integer=w426:i32)
                    }
                    frame #1 {
                      n273 = Less?(x=w435, y=0.0) -> (x < y?=w436:bool)
                      n274 = case shown="False" w436 {
                        tunnel: [FALSE w478] -> w437
                        tunnel: w435 -> [w439 _]
                        tunnel: [w439 0] -> w434
                        frame False {
                          n275 = flat-sequence {
                            frame #0 {
                              n276 = local read "Igniter Temp (°C)"() -> (w444:string)
                              n277 = Fract/Exp String To Number(string=w444) -> (number=w443:dbl)  [unwired: 3 in, 1 out]
                              n278 = Greater?(x="Igniter Minimum\nTemp (°C)", y=w443) -> (0:→"Igniter Abort":bool)
                            }
                            frame #1 {
                              n279 = local read "Countdown"() -> (w453:dbl)
                              n280 = local read "Elapsed Time"() -> (w450:u32)
                              n281 = Multiply(x=w453, y=-1000.0) -> (x*y=w451:dbl)
                              n282 = Multiply(x="Igniter Start", y=-1000.0) -> (x*y=w446:dbl)
                              n283 = Subtract(x=w451, y=w450) -> (x-y=w447:dbl)
                              n284 = Less?(x=w447, y=w446) -> (x < y?=w445:bool)
                              n285 = local write "Igniter Pwr"(w445) -> ()
                              n286 = case shown="True" w445 {
                                frame False {
                                }
                                frame True {
                                n287 = local read "Relay States"() -> (w455:bool[])
                                n288 = call "ADAM 5000 Relay Control.vi"("Relay States IN"=w455, "State"=TRUE, "Relay # (1=1st relay)"=15) -> ("Relay States OUT"=w454:bool[])  [unwired: 8 in]
                                n289 = local write "Relay States"(w454) -> ()
                                }
                              }
                            }
                            frame #2 {
                              n290 = local read "Countdown"() -> (w460:dbl)
                              n291 = local read "Elapsed Time"() -> (w463:u32)
                              n292 = Multiply(x=w460, y=-1000.0) -> (x*y=w462:dbl)
                              n293 = Multiply(x="MV Open Start", y=-1000.0) -> (x*y=w466:dbl)
                              n294 = Subtract(x=w462, y=w463) -> (x-y=w465:dbl)
                              n295 = Less?(x=w465, y=w466) -> (x < y?=w458:bool)
                              n296 = case shown="True" w458 {
                                frame False {
                                }
                                frame True {
                                n297 = local read "Igniter Abort"() -> (w470:bool)
                                n298 = Not(x="Sequence Abort") -> (.not. x?=w469:bool)
                                n299 = Not(x=w470) -> (.not. x?=w468:bool)
                                n300 = And(x=w469, y=w468) -> (x .and. y?=w467:bool)
                                n301 = case shown="True" w467 {
                                frame False {
                                }
                                frame True {
                                w472 = TRUE ("State")
                                n302 = local read "Relay States"() -> (w474:bool[])
                                n303 = local write "MV Open"(w472) -> ()
                                n304 = call "ADAM 5000 Relay Control.vi"("Relay States IN"=w474, "State"=w472, "Relay # (1=1st relay)"=6) -> ("Relay States OUT"=w473:bool[])  [unwired: 8 in]
                                n305 = local write "Relay States"(w473) -> ()
                                }
                                }
                                }
                              }
                            }
                          }
                        }
                        frame True {
                          n306 = local read "MV Open"() -> (w476:bool)
                          n307 = case shown="True" w476 {
                            tunnel: [w479 w485] -> w478
                            frame False {
                              n308 = flat-sequence {
                                tunnel: [TRUE] -> w479
                                frame #0 {
                                }
                                frame #1 {
                                n309 = local write "Auto Sequence"(FALSE ("Auto Sequence Flag")) -> ()
                                n310 = local write "Auto Sequence Flag"(FALSE ("Auto Sequence Flag")) -> ()
                                }
                                frame #2 {
                                }
                              }
                            }
                            frame True {
                              n311 = flat-sequence {
                                tunnel: [TRUE] -> w484
                                tunnel: w484 -> [w518]
                                tunnel: [w518] -> w483
                                tunnel: [w520] -> w485
                                tunnel: w483 -> [w520]
                                frame #0 {
                                n312 = Tick Count (ms)() -> (millisecond timer value=w486:u32)
                                n313 = while {
                                tunnel: "Burn Time" -> [w492]
                                tunnel: w486 -> [w497]
                                stop <- w493 stop-if-true
                                n314 = Tick Count (ms)() -> (millisecond timer value=w498:u32)
                                n315 = Wait (ms)(milliseconds to wait=u32 100) -> ()  [unwired: 1 out]
                                n316 = Subtract(x=w498, y=w497) -> (x-y=w496:u32)
                                n317 = Divide(x=w496, y=u32 1000) -> (x/y=w491:dbl)
                                n318 = Greater?(x=w491, y=w492) -> (0:w494:bool)
                                n319 = Subtract(x=w492, y=w491) -> (x-y=w490:dbl)
                                n320 = case shown="True" w494 {
                                tunnel: [FALSE TRUE] -> w493
                                frame False {
                                }
                                frame True {
                                }
                                }
                                n321 = Number To Fractional String(number=w490, precision (6)=i16 3) -> (F-format string=→"Burn Time\nCountdown (secs)":string)  [unwired: 2 in]
                                }
                                }
                                frame #1 {
                                n322 = local read "Relay States"() -> (w504:bool[])
                                n323 = call "ADAM 5000 Relay Control.vi"("Relay States IN"=w504, "State"=FALSE, "Relay # (1=1st relay)"=12) -> ("Relay States OUT"=w505:bool[])  [unwired: 8 in]
                                n324 = local write "Relay States"(w505) -> ()
                                }
                                frame #2 {
                                w508 = FALSE ("Auto Sequence Flag")
                                w507 = TRUE ("State")
                                n325 = local read "Relay States"() -> (w511:bool[])
                                n326 = local write "Auto Sequence Flag"(FALSE ("Auto Sequence Flag")) -> ()
                                n327 = local write "MV Open"(w508) -> ()
                                n328 = local write "Auto Sequence"(w508) -> ()
                                n329 = local write "Burn Time\nCountdown (secs)"("0.000" ("Burn Time\nCountdown (secs)")) -> ()
                                n330 = local write "MV Closed"(w507) -> ()
                                n331 = call "ADAM 5000 Relay Control.vi"("Relay States IN"=w511, "State"=w507, "Relay # (1=1st relay)"=13) -> ("Relay States OUT"=w512:bool[])  [unwired: 8 in]
                                n332 = local write "Relay States"(w512) -> ()
                                }
                                frame #3 {
                                w514 = FALSE ("State")
                                n333 = local read "Relay States"() -> (w516:bool[])
                                n334 = local write "Igniter Pwr"(w514) -> ()
                                n335 = call "ADAM 5000 Relay Control.vi"("Relay States IN"=w516, "State"=w514, "Relay # (1=1st relay)"=15) -> ("Relay States OUT"=w515:bool[])  [unwired: 8 in]
                                n336 = local write "Relay States"(w515) -> ()
                                }
                                frame #4 {
                                n337 = Wait (ms)(milliseconds to wait=u32 2000) -> ()  [unwired: 1 out]
                                }
                              }
                            }
                          }
                        }
                      }
                    }
                    frame #2 {
                      "Countdown (secs)" <- w521
                    }
                  }
                  n338 = Wait (ms)(milliseconds to wait=u32 100) -> ()  [unwired: 1 out]
                }
              }
            }
          }
        }
      }
    }
    n339 = local read "stop"() -> (w398:bool)
  }
